vi "Make DLL Param(Read Batch Profile Req).vi"(1 "Read Batch Profile Req":T3={"Read Area"=TRUE, "Batch Pos"=0, "Read Batch No"=0, "Read Profile No."=0, "Read Profile Cnt"=0, "Erase"=FALSE} {"Batch Pos" items=["CURRENT"=0, "SPECIFY"=2, "COMMITED"=3, "NEWEST PROFILE"=4]}) -> (0 "pReq":T2 {"Batch Pos" items=["CURRENT"=0, "SPECIFY"=2, "COMMITED"=3, "NEWEST PROFILE"=4]})   [LabVIEW 2014, in "Keyence LJ-V7000.lvlib"]
uses:
  Keyence LJ-V7000.lvlib
  Public/Clusters/Read Batch Profile Req.ctl
  Public/constant/Batch Pos.ctl
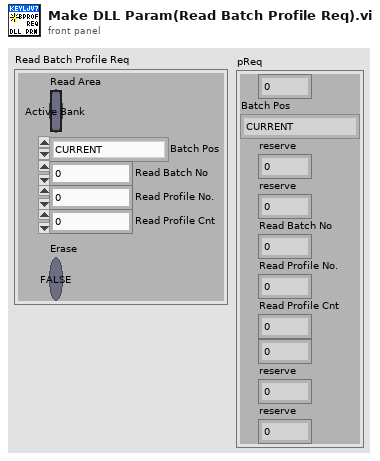
[diagram p1: front panel]
types:
  T1 = typedef "Keyence LJ-V7000.lvlib/Batch Pos.ctl" = u8
  T2 = cluster{u8, "Batch Pos":T1, "reserve":u8, "reserve":u8, "Read Batch No":u32, "Read Profile No.":u32, "Read Profile Cnt":u8, u8, "reserve":u8, "reserve":u8}
  T3 = typedef "Keyence LJ-V7000.lvlib/Read Batch Profile Req.ctl" = cluster{"Read Area":bool, "Batch Pos":T1, "Read Batch No":u32, "Read Profile No.":u32, "Read Profile Cnt":u8, "Erase":bool}
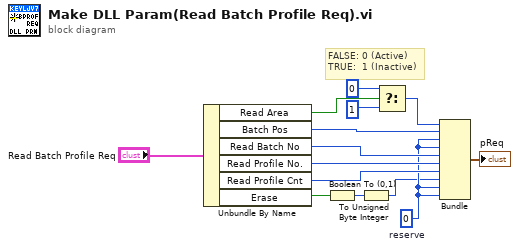
[diagram p0: block diagram]
diagram:
  w4 = u8 0  # reserve
  # "FALSE: 0 (Active)\nTRUE:  1 (Inactive)"
  n1 = Unbundle By Name("Read Batch Profile Req") -> ("Read Area"=w14:bool, "Batch Pos"=w10:T1, "Read Batch No"=w9:u32, "Read Profile No."=w8:u32, "Read Profile Cnt"=w5:u8, "Erase"=w3:bool)
  n2 = Boolean To (0,1)(Boolean=w3) -> (0, 1=w7:i16)
  n3 = To Unsigned Byte Integer(number=w7) -> (unsigned 8bit integer=w2:u8)
  n4 = Select(t=u8 0, s=w14, f=u8 1) -> (s? t:f=w11:u8)
  n5 = Bundle(w11, "Batch Pos"=w10, "reserve"=w4, "reserve"=w4, "Read Batch No"=w9, "Read Profile No."=w8, "Read Profile Cnt"=w5, w2, "reserve"=w4, "reserve"=w4) -> (→"pReq":T2)  [unwired: 1 in]
